vi "Write to network variable.vi"(8 "error in (no error)":errorcluster, 11 "created path":path) -> (0 "error out":errorcluster, 3 "created path (dup)":path)   [LabVIEW 2013]
uses:
  Global Variables/General Globals.vi
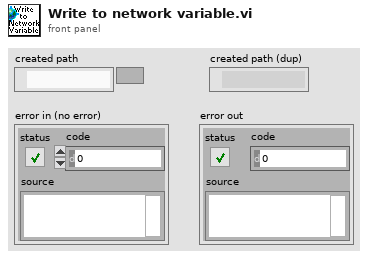
[diagram p1: front panel]
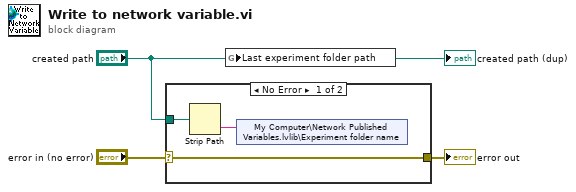
[diagram p0: block diagram]
diagram:
  n1 = case shown="No Error" "error in (no error)" {
    selector: "error in (no error)" -> [w5 w7]
    tunnel: "created path" -> [w6 _]
    tunnel: [w5 w7] -> w3
    frame No Error {
      n2 = Strip Path(path=w6) -> (name=w4:string)  [unwired: 1 out]
      n3 = shared-variable "My Computer\\Network Published Variables.lvlib\\Experiment folder name"(w4) -> ()  [unwired: 1 in, 1 out]
    }
    frame Error {
    }
  }
  "error out" <- w3
  n4 = global write "General Globals.vi" "Last experiment folder path"("created path") -> ()
  "created path (dup)" <- "created path"
